vi "BDSyringeHelper.vi"(0 "object in":refnum<class "CetoniPump.lvclass">, 2 "Syringe":T2(ring), 5 "error in (no error)":errorcluster) -> (14 "object out":refnum<class "CetoniPump.lvclass">, 16 "output cluster":T1, 19 "error out":errorcluster)   [LabVIEW 2021, in "CetoniPump.lvclass"]
uses:
  CetoniPump.lvclass
  CetoniPump.lvclass/CetoniPump.ctl
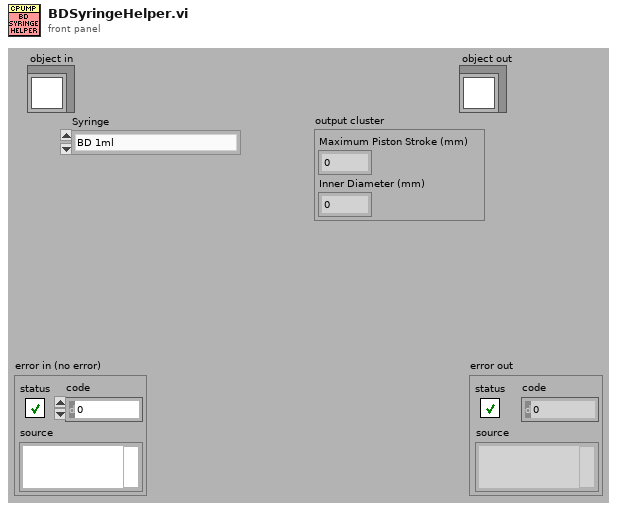
[diagram p1: front panel]
types:
  T1 = cluster{"Maximum Piston Stroke (mm)":dbl, "Inner Diameter (mm)":dbl}
  T2 = enum16{"BD 1ml", "BD 3ml", "BD 5ml", "BD 10ml", "BD 20ml", "BD 30ml", "BD 50ml", "HSW 1ml"}
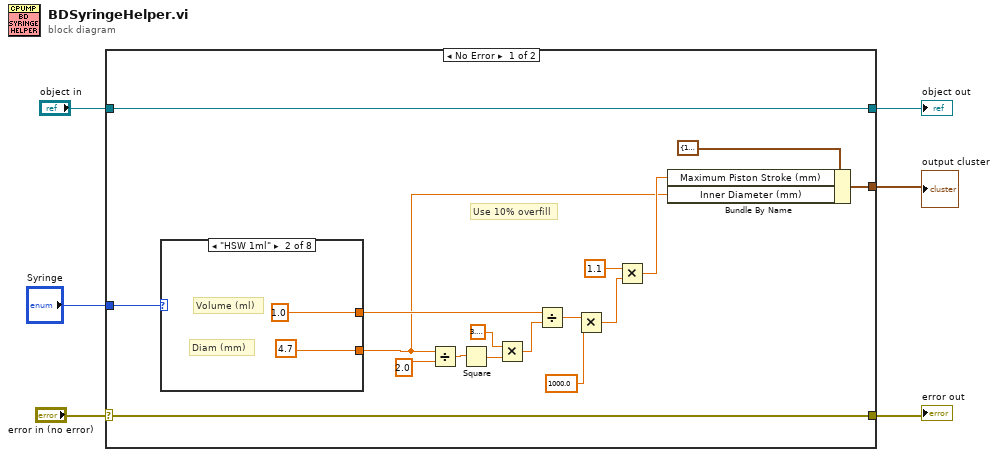
[diagram p0: block diagram]
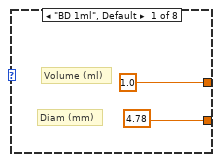
[diagram p2: hidden frame]
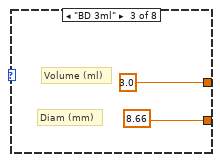
[diagram p3: hidden frame]
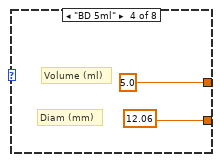
[diagram p4: hidden frame]
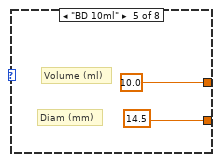
[diagram p5: hidden frame]
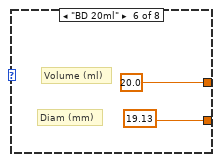
[diagram p6: hidden frame]
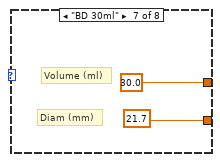
[diagram p7: hidden frame]
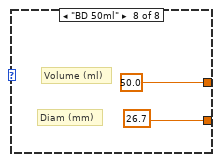
[diagram p8: hidden frame]
diagram:
  n1 = case shown="No Error" "error in (no error)" {
    selector: "error in (no error)" -> [w23 w41]
    tunnel: [w23 w41] -> w5
    tunnel: [w22 w40] -> w3
    tunnel: "object in" -> [w22 w40]
    tunnel: [w8 _] -> w2
    tunnel: "Syringe" -> [w7 _]
    frame No Error {
      # "Use 10% overfill"
      n2 = case shown="\"HSW 1ml\"" w7 {
        tunnel: [1.0 1.0 3.0 5.0 10.0 20.0 30.0 50.0] -> w15
        tunnel: [4.78 4.7 8.66 12.06 14.5 19.13 21.7 26.7] -> w9
        frame "BD 1ml", Default {
          # "Diam (mm)"
          # "Volume (ml)"
        }
        frame "HSW 1ml" {
          # "Diam (mm)"
          # "Volume (ml)"
        }
        frame "BD 3ml" {
          # "Diam (mm)"
          # "Volume (ml)"
        }
        frame "BD 5ml" {
          # "Diam (mm)"
          # "Volume (ml)"
        }
        frame "BD 10ml" {
          # "Diam (mm)"
          # "Volume (ml)"
        }
        frame "BD 20ml" {
          # "Diam (mm)"
          # "Volume (ml)"
        }
        frame "BD 30ml" {
          # "Diam (mm)"
          # "Volume (ml)"
        }
        frame "BD 50ml" {
          # "Diam (mm)"
          # "Volume (ml)"
        }
      }
      n3 = Divide(x=w9, y=2.0) -> (x/y=w20:dbl)
      n4 = Square(x=w20) -> (x^2=w19:dbl)
      n5 = Multiply(x=3.141592653589793, y=w19) -> (x*y=w16:dbl)
      n6 = Divide(x=w15, y=w16) -> (x/y=w13:dbl)
      n7 = Multiply(x=w13, y=1000.0) -> (x*y=w12:dbl)
      n8 = Multiply(x=1.1, y=w12) -> (x*y=w10:dbl)
      n9 = Bundle By Name(cluster=T1 {"Maximum Piston Stroke (mm)"=100.0, "Inner Diameter (mm)"=12.0} ("SyringeSettings"), "Maximum Piston Stroke (mm)"=w10, "Inner Diameter (mm)"=w9) -> (w8:T1)
    }
    frame Error {
    }
  }
  "error out" <- w5
  "object out" <- w3
  "output cluster" <- w2
